vi "Printer interface main.vi"(11 "Printer Interface":refnum<queue>) -> ()   [LabVIEW 2024]
uses:
  ARCH/Message Queue/Message Cluster.ctl
  CTRLS/Printer interface cluster.ctl
  CTRLS/Open Batch Data.ctl
  CTRLS/Printer Message settings.ctl
  CTRLS/GLB_VAR.vi
  ARCH/Message Queue/Message Queue.lvlib
panel:
  in  "Interface Cluster":T1
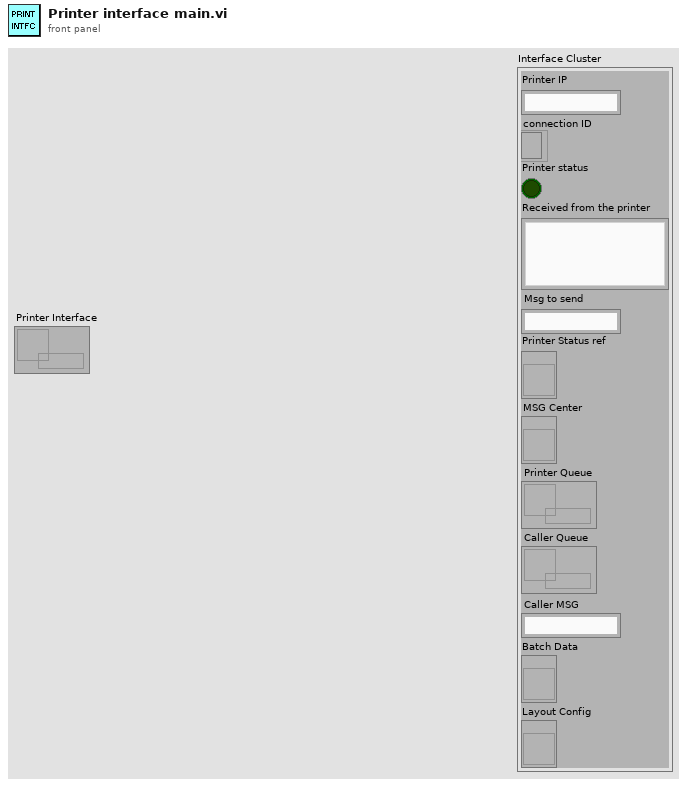
[diagram p1: front panel]
types:
  T1 = typedef "Printer interface cluster.ctl" = cluster{"Printer IP":string, "connection ID":refnum<k5>, "Printer status":bool, "Received from the printer":string, "Msg to send":string, "Printer Status ref":refnum<vi>, "MSG Center":refnum<vi>, "Printer Queue":refnum<queue>, "Caller Queue":refnum<queue>, "Caller MSG":string, "Batch Data":refnum<vi>, "Layout Config":refnum<vi>}
  T2 = typedef "Message Queue.lvlib/Message Cluster.ctl" = cluster{"Message":string, "Message Data":variant}
  T3 = typedef "REF.ctl" = cluster{"Save Settings":refnum<vi>, "Navigation":refnum<vi>, "Main Tab":refnum<vi>, "Password":refnum<vi>, "BatchData":refnum<vi>, "Serial Data":refnum<vi>, "Username":refnum<vi>, "Stop Printing":refnum<vi>, "Run statistics":refnum<vi>, "System settings":refnum<vi>, "Batch Managment contol":refnum<vi>, "Start Printing":refnum<vi>, "BatchData MNG":refnum<vi>, "MSG Cenetr":refnum<vi>, "Printer status":refnum<vi>, "Printer Message Config":refnum<vi>, "Ready and Paused Batches":refnum<vi>, "Camera Setup":refnum<vi>, "Batch statistics":refnum<vi>, "Logout":refnum<vi>}
  T4 = typedef "System settings.ctl" = cluster{"Machine IP":string, "Camera IP":string, "Printer IP":string, "Scanner settings":string, "Server Path":path, "Sending Port":u32, "Recieveing Port":u32}
  T5 = typedef "All Message Queues.ctl" = cluster{"DB":refnum<queue>, "Printer":refnum<queue>, "Camera":refnum<queue>, "Printer Interface":refnum<queue>, "WO":refnum<queue>}
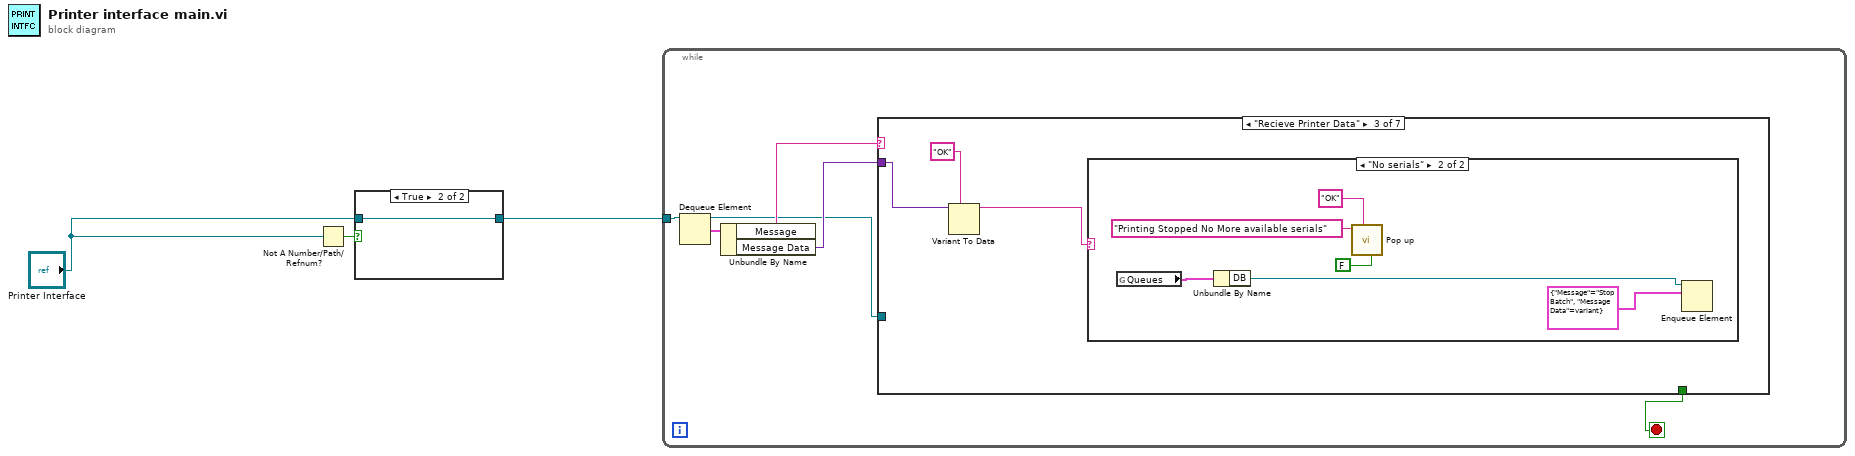
[diagram p0: block diagram]
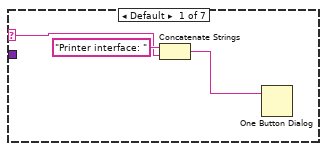
[diagram p3: hidden frame]
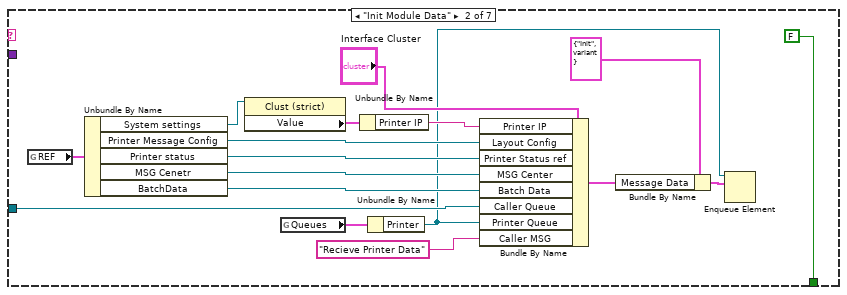
[diagram p4: hidden frame]
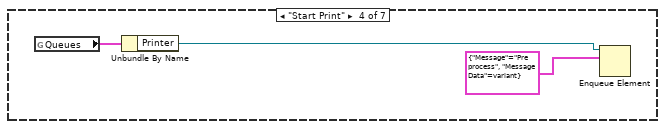
[diagram p6: hidden frame]
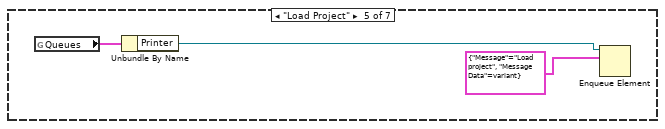
[diagram p7: hidden frame]
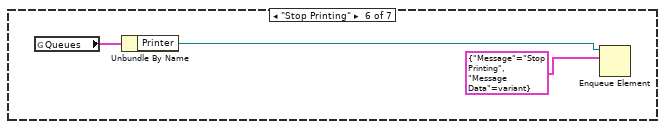
[diagram p8: hidden frame]
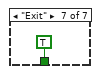
[diagram p9: hidden frame]
diagram:
  n1 = Not A Number/Path/Refnum?(number/path/refnum="Printer Interface") -> (NaN/Path/Refnum?=w2:bool)
  n2 = case shown="True" w2 {
    tunnel: [w4 w5] -> w1
    tunnel: "Printer Interface" -> [w4 w5]
    frame False {
    }
    frame True {
    }
  }
  n3 = while {
    tunnel: w1 -> [w11]
    stop <- w7 stop-if-true
    n4 = Dequeue Element(queue=w11) -> (queue out=w6:refnum<queue>, element=w10:T2)  [unwired: 2 in, 2 out]
    n5 = Unbundle By Name(w10) -> ("Message"=w9:string, "Message Data"=w8:variant)
    n6 = case shown="\"Recieve Printer Data\"" w9 {
      selector: w9 -> [w12 _ _ _ _ _ _]
      tunnel: w8 -> [_ _ w32 _ _ _ _]
      tunnel: [_ FALSE _ _ _ _ TRUE] -> w7
      tunnel: w6 -> [_ w21 _ _ _ _ _]
      frame Default {
        n7 = Concatenate Strings("Printer interface: " ("string"), w12) -> (w13:string)
        n8 = One Button Dialog(message=w13) -> ()  [unwired: 1 in, 1 out]
      }
      frame "Init Module Data" {
        n9 = global read "GLB_VAR.vi" "REF"() -> (w29:T3)
        n10 = Unbundle By Name(w29) -> ("System settings"=w28:refnum<vi>, "Printer Message Config"=w25:refnum<vi>, "Printer status"=w24:refnum<vi>, "MSG Cenetr"=w23:refnum<vi>, "BatchData"=w22:refnum<vi>)
        n11 = property class="Clust (strict)"(reference=w28) -> ("Value"=w27:T4)  [unwired: 1 in, 2 out]
        n12 = global read "GLB_VAR.vi" "Queues"() -> (w20:T5)
        n13 = Unbundle By Name(w27) -> ("Printer IP"=w26:string)
        n14 = Unbundle By Name(w20) -> ("Printer"=w18:refnum<queue>)
        n15 = Bundle By Name(cluster="Interface Cluster", "Printer IP"=w26, "Layout Config"=w25, "Printer Status ref"=w24, "MSG Center"=w23, "Batch Data"=w22, "Caller Queue"=w21, "Printer Queue"=w18, "Caller MSG"="Recieve Printer Data") -> (w16:T1)
        n16 = Bundle By Name(cluster=T2 {"Message"="Init", "Message Data"=variant} ("element"), "Message Data"=w16) -> (w15:T2)
        n17 = Enqueue Element(queue=w18, element=w15) -> ()  [unwired: 2 in, 3 out]
      }
      frame "Recieve Printer Data" {
        n18 = Variant To Data(type="OK" ("OK Boolean Text"), Variant=w32) -> (data=w33:string)  [unwired: 1 in, 1 out]
        n19 = case shown="\"No serials\"" w33 {
          frame "False", Default {
          }
          frame "No serials" {
            n20 = global read "GLB_VAR.vi" "Queues"() -> (w37:T5)
            n21 = Unbundle By Name(w37) -> ("DB"=w36:refnum<queue>)
            n22 = call "Pop up.vi"("Close Visible"=FALSE, "OK Boolean Text"="OK", "Title IN"="Printing Stopped No More available serials") -> ()  [unwired: 7 in, 2 out]
            n23 = Enqueue Element(queue=w36, element=T2 {"Message"="Stop Batch", "Message Data"=variant}) -> ()  [unwired: 2 in, 3 out]
          }
        }
      }
      frame "Start Print" {
        n24 = global read "GLB_VAR.vi" "Queues"() -> (w43:T5)
        n25 = Unbundle By Name(w43) -> ("Printer"=w42:refnum<queue>)
        n26 = Enqueue Element(queue=w42, element=T2 {"Message"="Pre process", "Message Data"=variant}) -> ()  [unwired: 2 in, 3 out]
      }
      frame "Load Project" {
        n27 = global read "GLB_VAR.vi" "Queues"() -> (w46:T5)
        n28 = Unbundle By Name(w46) -> ("Printer"=w45:refnum<queue>)
        n29 = Enqueue Element(queue=w45, element=T2 {"Message"="Load project", "Message Data"=variant}) -> ()  [unwired: 2 in, 3 out]
      }
      frame "Stop Printing" {
        n30 = global read "GLB_VAR.vi" "Queues"() -> (w49:T5)
        n31 = Unbundle By Name(w49) -> ("Printer"=w48:refnum<queue>)
        n32 = Enqueue Element(queue=w48, element=T2 {"Message"="Stop Printing", "Message Data"=variant}) -> ()  [unwired: 2 in, 3 out]
      }
      frame "Exit" {
      }
    }
  }
